vi "Configure Parent Class.vi"(8 "error in (no error)":errorcluster, 10 "Parent Class":string, 11 "New Class Dialog In":refnum<class "New Class Dialog.lvclass">) -> (0 "error out":errorcluster, 3 "New Class Dialog Out":refnum<class "New Class Dialog.lvclass">)   [LabVIEW 2020, in "New Class Dialog.lvclass"]
uses:
  New Class Dialog.lvclass
  Framework/Process/Process.lvclass
  Framework Test/Process Test/Process Test.lvclass
  C:/Program Files (x86)/National Instruments/LabVIEW 2020/vi.lib/Asteme/LUnit/Test Case.lvclass
  New Class Dialog.lvclass/New Class Dialog.ctl
  Class Generation/Process Generator/Process Generator.lvclass/Process Generator.ctl
  Class Generation/Process Generator/Process Generator.lvclass
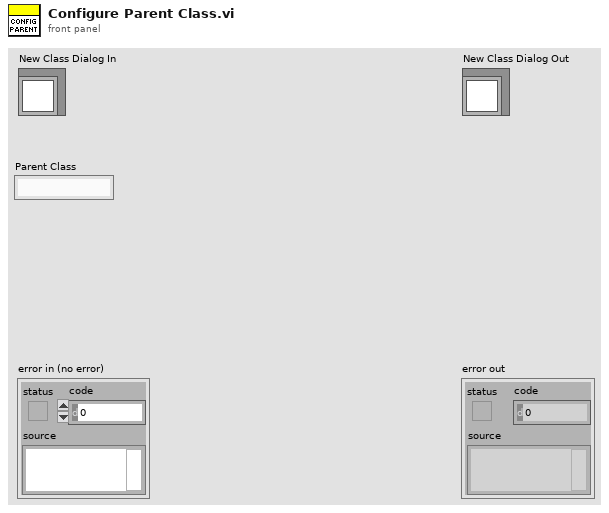
[diagram p1: front panel]
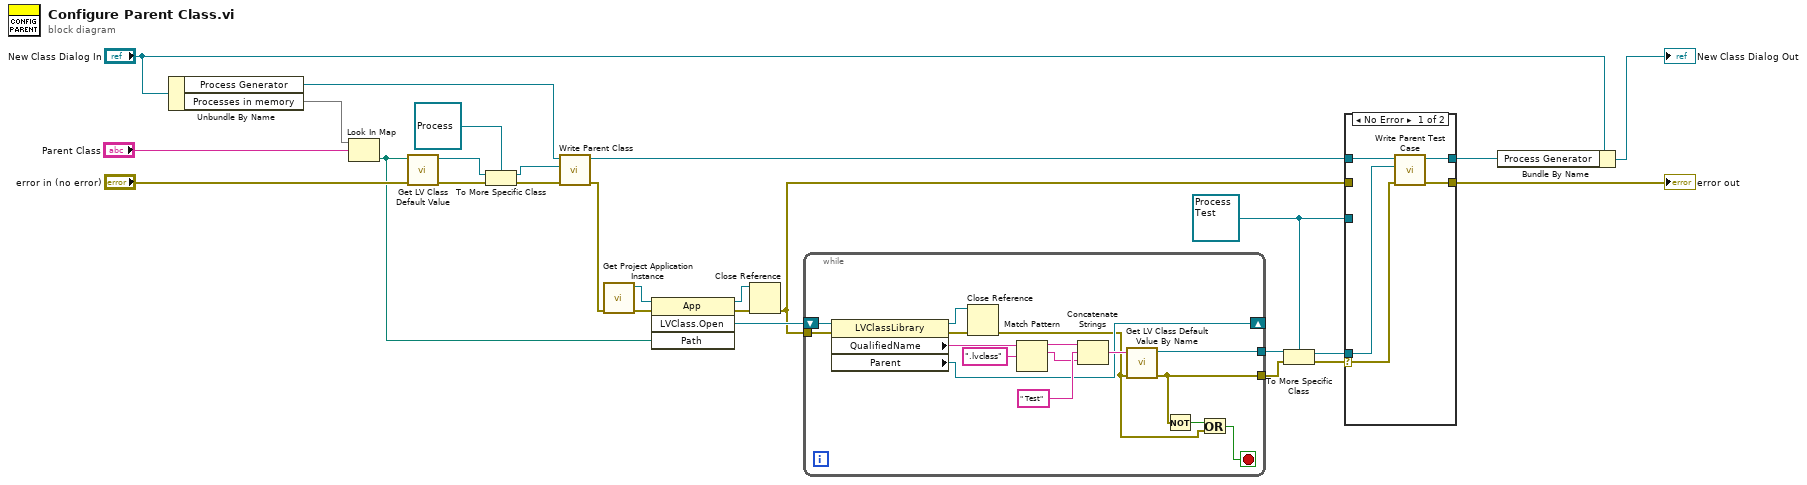
[diagram p0: block diagram]
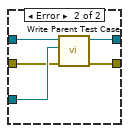
[diagram p2: hidden frame]
diagram:
  w2 = refnum<class "Process Test.lvclass"> refnum ("Process Test.lvclass")
  n1 = Unbundle By Name("New Class Dialog In") -> ("Process Generator"=w19:refnum<class "Process Generator.lvclass">, "Processes in memory"=w27:map{string, path})
  n2 = Look In Map(map=w27, key="Parent Class") -> (value=w16:path)  [unwired: 1 in, 1 out]
  n3 = call <vilib>:"Get LV Class Default Value.vi"("error in (no error)"="error in (no error)", "class path"=w16) -> ("error out"=w21:errorcluster, "object"=w23:refnum<class>)  [unwired: 8 in]
  n4 = To More Specific Class(target class=refnum<class "Process.lvclass"> refnum ("Parent Process"), reference=w23, error in=w21) -> (specific class reference=w25:refnum<class "Process.lvclass">, error out=w20:errorcluster)
  n5 = call "Write Parent Class.vi"("error in (no error)"=w20, "Parent Process"=w25, "Process Generator in"=w19) -> ("error out"=w10:errorcluster, "Process Generator out"=w8:refnum<class "Process Generator.lvclass">)  [unwired: 7 in]
  n6 = call "Get Project Application Instance.vi"("error in (no error)"=w10) -> ("error out"=w14:errorcluster, "Application out"=w15:refnum<vi>)  [unwired: 9 in]
  n7 = invoke class="App" method="LVClass.Open"(reference=w15, error in=w14, "Path"=w16) -> (reference out=w11:refnum<vi>, error out=w12:errorcluster, "LVClass.Open"=w13:refnum<vi>)  [unwired: 1 in, 1 out]
  n8 = Close Reference(reference=w11, error in (no error)=w12) -> (error out=w1:errorcluster)
  n9 = while {
    tunnel: w1 -> [w42]
    tunnel: [w33] -> w9
    shift-right: [w32] -> _
    shift-left: w13 -> [w43]
    tunnel: [w28] -> w4
    stop <- w31 stop-if-true
    n10 = property class="LVClassLibrary"(reference=w43, error in=w42) -> (reference out=w34:refnum<vi>, error out=w35:errorcluster, "QualifiedName"=w41:string, "Parent"=w32:refnum<vi>)
    n11 = Close Reference(reference=w34, error in (no error)=w35) -> (error out=w29:errorcluster)
    n12 = Match Pattern(string=w41, regular expression=".lvclass") -> (before substring=w39:string, match substring=w37:string)  [unwired: 1 in, 2 out]
    n13 = Concatenate Strings(w39, " Test" ("string"), w37) -> (w36:string)
    n14 = call <vilib>:"Get LV Class Default Value By Name.vi"("error in (no error)"=w29, "class name"=w36) -> ("error out"=w28:errorcluster, "object"=w33:refnum<class>)  [unwired: 8 in]
    n15 = Not(x=w28) -> (.not. x?=w30:bool)
    n16 = Or(x=w30, y=w29) -> (x .or. y?=w31:bool)
  }
  n17 = To More Specific Class(target class=w2, reference=w9, error in=w4) -> (specific class reference=w6:refnum<class "Process Test.lvclass">, error out=w5:errorcluster)
  n18 = case shown="No Error" w5 {
    selector: w5 -> [w45 _]
    tunnel: w8 -> [w48 w53]
    tunnel: [w47 w52] -> w7
    tunnel: w6 -> [w46 _]
    tunnel: [w44 w51] -> w3
    tunnel: w2 -> [_ w50]
    tunnel: w1 -> [_ w49]
    frame No Error {
      n19 = call "Write Parent Test Case.vi"("error in (no error)"=w45, "Parent Test Case"=w46, "Process Generator In"=w48) -> ("error out"=w44:errorcluster, "Process Generator Out"=w47:refnum<class "Process Generator.lvclass">)  [unwired: 7 in]
    }
    frame Error {
      n20 = call "Write Parent Test Case.vi"("error in (no error)"=w49, "Parent Test Case"=w50, "Process Generator In"=w53) -> ("error out"=w51:errorcluster, "Process Generator Out"=w52:refnum<class "Process Generator.lvclass">)  [unwired: 7 in]
    }
  }
  "error out" <- w3
  n21 = Bundle By Name(cluster="New Class Dialog In", "Process Generator"=w7) -> (→"New Class Dialog Out":refnum<class "New Class Dialog.lvclass">)
